vi "Initialize.vi"(6 "timeout in ms":i32=30000, 7 "Engine Configuration":refnum<class "engine configuration.lvclass">, 8 "error in":errorcluster, 9 "Module Configurations":refnum<class "TBM module configuration.lvclass">[](array[class]), 10 "Modules":refnum<class "TBM module execution interface.lvclass">[](array[class]), 11 "Standard Engine Runtime in":refnum<class "Standard Engine Runtime.lvclass">) -> (0 "error out":errorcluster, 3 "Standard Engine Runtime out":refnum<class "Standard Engine Runtime.lvclass">)   [LabVIEW 2013, in "Standard Engine Runtime.lvclass"]
doc: "This VI passes all the information necessary for initializing an engine to the engine background process. That backround process will then initialize itself as well as all of the modules it will be interacting with."
uses:
  Standard Engine Runtime.lvclass
  <vilib>/NI/Tag Bus Module Framework/module configuration/TBM module configuration.lvclass
  <vilib>/NI/Tag Bus Module Framework/runtime/TBM module execution interface.lvclass
  <vilib>/NI/Module Execution Interface/Engine Configuration/engine configuration.lvclass
  Configuration/Standard Engine Configuration.lvclass
  <vilib>/NI/Module Execution Interface/Engine Runtime/Execution States.ctl
  Standard Engine Runtime.lvclass/Standard Engine Runtime.ctl
  <vilib>/NI/Module Execution Interface/Engine Runtime/Engine Runtime Interface.lvclass
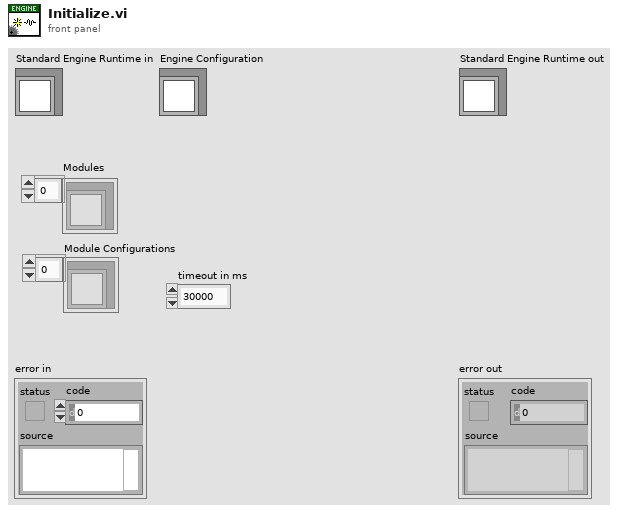
[diagram p1: front panel]
types:
  T1 = typedef "main engine.lvlib/Engine Data.ctl" = cluster{"timed loop timer source":T2, "control loop data":T3, "status reporting":T15}
  T2 = typedef "main engine.lvlib/timed loop timing sources.ctl" = cluster{"Processor":i32, "Priority":i32, "timing source dt":u32, "timer source":refnum<class "TBM timing source.lvclass">}
  T3 = typedef "main engine.lvlib/control loop data.ctl" = cluster{"engine tag bus":T4, "engine schedule":T5, "module information":T7[]}
  T4 = typedef "tag bus.lvlib/data table.lvlib/data table.ctl" = cluster{"Double":dbl[], "Single":sgl[], "I64":i64[], "I32":i32[], "I16":i16[], "I8":i8[], "U64":u64[], "U32":u32[], "U16":u16[], "U8":u8[], "Boolean":bool[], "String":string[], "Array of Double":cluster{"DBL Array":dbl[]}[], "Array of Single":cluster{"SGL Array":sgl[]}[], "Array of I64":cluster{"I64 Array":i64[]}[], "Array of I32":cluster{"I32 Array":i32[]}[], "Array of I16":cluster{"I16 Array":i16[]}[], "Array of I8":cluster{"I8 Array":i8[]}[], "Array of U64":cluster{"U64 Array":u64[]}[], "Array of U32":cluster{"U32 Array":u32[]}[], "Array of U16":cluster{"U16 Array":u16[]}[], "Array of U8":cluster{"U8 Array":u8[]}[], "Array of Boolean":cluster{"Boolean Array":bool[]}[], "Array of String":cluster{"String Array":string[]}[]}
  T5 = typedef "main engine.lvlib/engine run schedule.ctl" = cluster{"module run flags":u8[], "decimation schedule":T6}
  T6 = typedef "main engine.lvlib/engine decimation schedule.ctl" = cluster{"decimations":u16[], "offsets":u16[]}
  T7 = typedef "main engine.lvlib/full module data.ctl" = cluster{"run state":T8, "module":refnum<class "TBM module execution interface.lvclass">, "module ref":refnum<data-value>, "async exec ref":T9, "configuration ref":refnum<data-value>, "error":errorcluster, "previous error code":i32, "input method":T10, "output method":T10, "process method parameters":T10, "process method results":T10, "fault handling":T13, "error report index ":i32}
  T8 = typedef "main engine.lvlib/module run state.ctl" = enum16{"sync", "async"}
  T9 = typedef "async executor.lvlib/asynchronous executor reference.ctl" = cluster{"command fifo":refnum<k33>, "error fifo":refnum<k33>, "VI Refnum":refnum<vi>, "input buffer":refnum<k33>, "output buffer":refnum<k33>, "process buffer":refnum<k33>, "original dvrs":refnum<data-value>[]}
  T10 = typedef "main engine.lvlib/module method data.ctl" = cluster{"data table":T4, "transfer spec":T11[]}
  T11 = typedef "tag bus.lvlib/data table.lvlib/transfer specification.ctl" = cluster{"data type":T12, "sink indices":i32[], "source indices":i32[]}
  T12 = typedef "tag bus.lvlib/tag descriptor.lvclass/Data Type.ctl" = enum16{"Double", "Single", "I64", "I32", "I16", "I8", "U64", "U32", "U16", "U8", "Boolean", "String", "Array of Double", "Array of Single", "Array of I64", "Array of I32", "Array of I16", "Array of I8", "Array of U64", "Array of U32", "Array of U16", "Array of U8", "Array of Boolean", "Array of String"}
  T13 = typedef "main engine.lvlib/fault handling spec.ctl" = cluster{"unknown":T14[], "trivial":T14[], "critical":T14[], "recoverable":T14[]}
  T14 = typedef "Standard Engine Configuration.lvclass/Error Actions.ctl" = enum16{"Clear", "Notify", "Stop Component", "Stop Engine", "Safe State", "Attempt Recovery"}
  T15 = typedef "main engine.lvlib/status reporting data.ctl" = cluster{"late? index (bool)":i32, "late count index (U32)":i32, "dt (ns) index (U64)":i32}
  T16 = typedef "Engine Runtime Interface.lvclass/Execution States.ctl" = enum16{"Init", "Pre-Operational", "Safe-Operational", "Operational", "Stopped"}
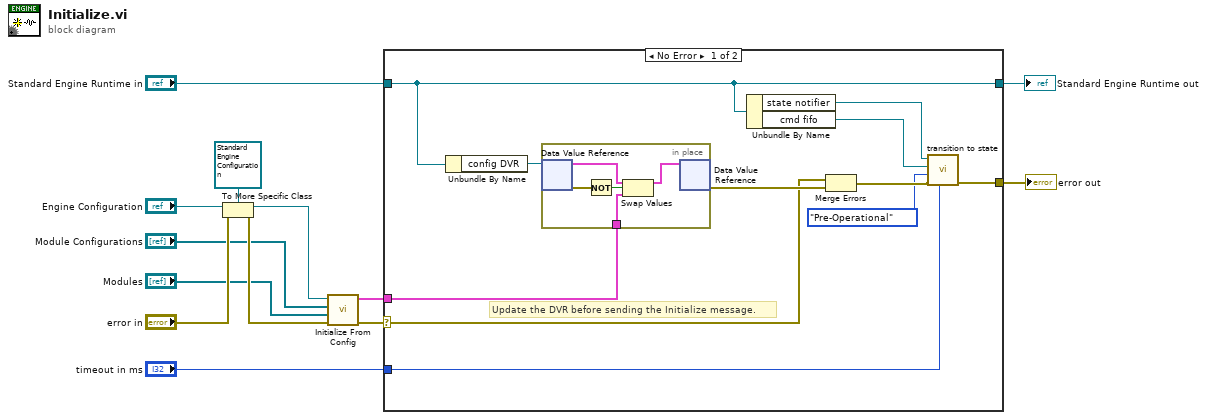
[diagram p0: block diagram]
diagram:
  n1 = To More Specific Class(target class=refnum<class "Standard Engine Configuration.lvclass"> refnum ("Engine Configuration"), reference="Engine Configuration", error in="error in") -> (specific class reference=w4:refnum<class "Standard Engine Configuration.lvclass">, error out=w6:errorcluster)
  n2 = call "Initialize From Config.vi"("error in"=w6, "Modules"="Modules", "Module Configurations"="Module Configurations", "Engine Configuration"=w4) -> ("error out"=w5:errorcluster, "Engine Data Out"=w1:T1)  [unwired: 6 in]
  n3 = case shown="No Error" w5 {
    selector: w5 -> [w22 w31]
    tunnel: "Standard Engine Runtime in" -> [w20 w30]
    tunnel: "timeout in ms" -> [w19 _]
    tunnel: [w18 w31] -> w8
    tunnel: [w20 w30] -> w7
    tunnel: w1 -> [w21 _]
    frame No Error {
      # "Update the DVR before sending the Initialize message."
      n4 = Unbundle By Name(w20) -> ("config DVR"=w24:refnum<data-value>)
      n5 = in-place {
        in-place-border: w21 -> [w25]
        n6 = in-place-dvr #1(w24) -> (w27:T1, w29:errorcluster)
        n7 = Not(x=w29) -> (.not. x?=w28:bool)
        n8 = Swap Values(12:w27, 13:w28, 14:w25) -> (1:w26:T1)  [unwired: 1 out]
        n9 = in-place-dvr #1(w26) -> (w23:errorcluster)  [unwired: 1 out]
      }
      n10 = Unbundle By Name(w20) -> ("state notifier"=w16:refnum<notifier>, "cmd fifo"=w15:refnum<k33>)
      n11 = Merge Errors(w22, w23) -> (w17:errorcluster)
      n12 = call "transition to state.vi"("timeout"=w19, "error in"=w17, "States"=Execution_States."Pre-Operational" ("element"), "cmd fifo"=w15, "notifier"=w16) -> ("error out"=w18:errorcluster)  [unwired: 6 in]
    }
    frame Error {
    }
  }
  "error out" <- w8
  "Standard Engine Runtime out" <- w7
